vi "LoadFeedforward.vi"(8 "error in":errorcluster, 10 "show ref":refnum<vi>, 11 "Path":path) -> (0 "error out":errorcluster, 2 "values Q":dbl[](array[numeric]), 3 "values I":dbl[](array[numeric]))   [LabVIEW 2013]
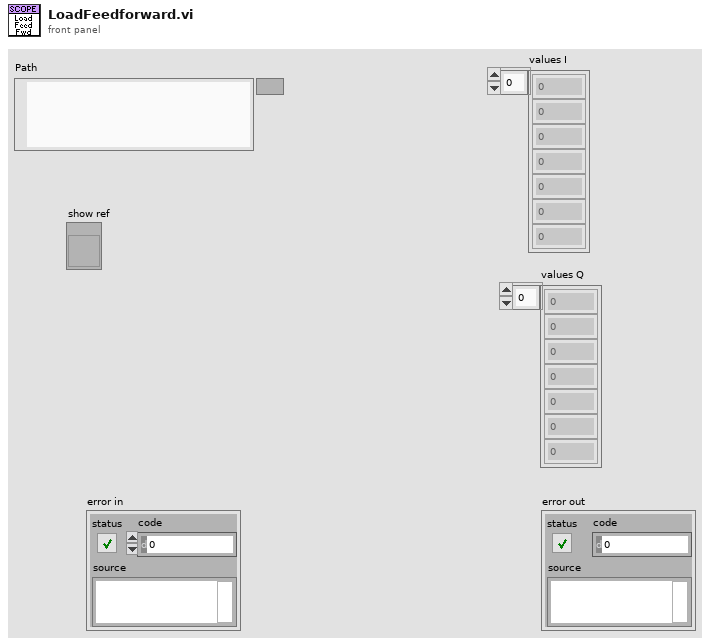
[diagram p1: front panel]
types:
  T1 = enum8{"Enabled", "Disabled", "Disabled and Grayed Out"}
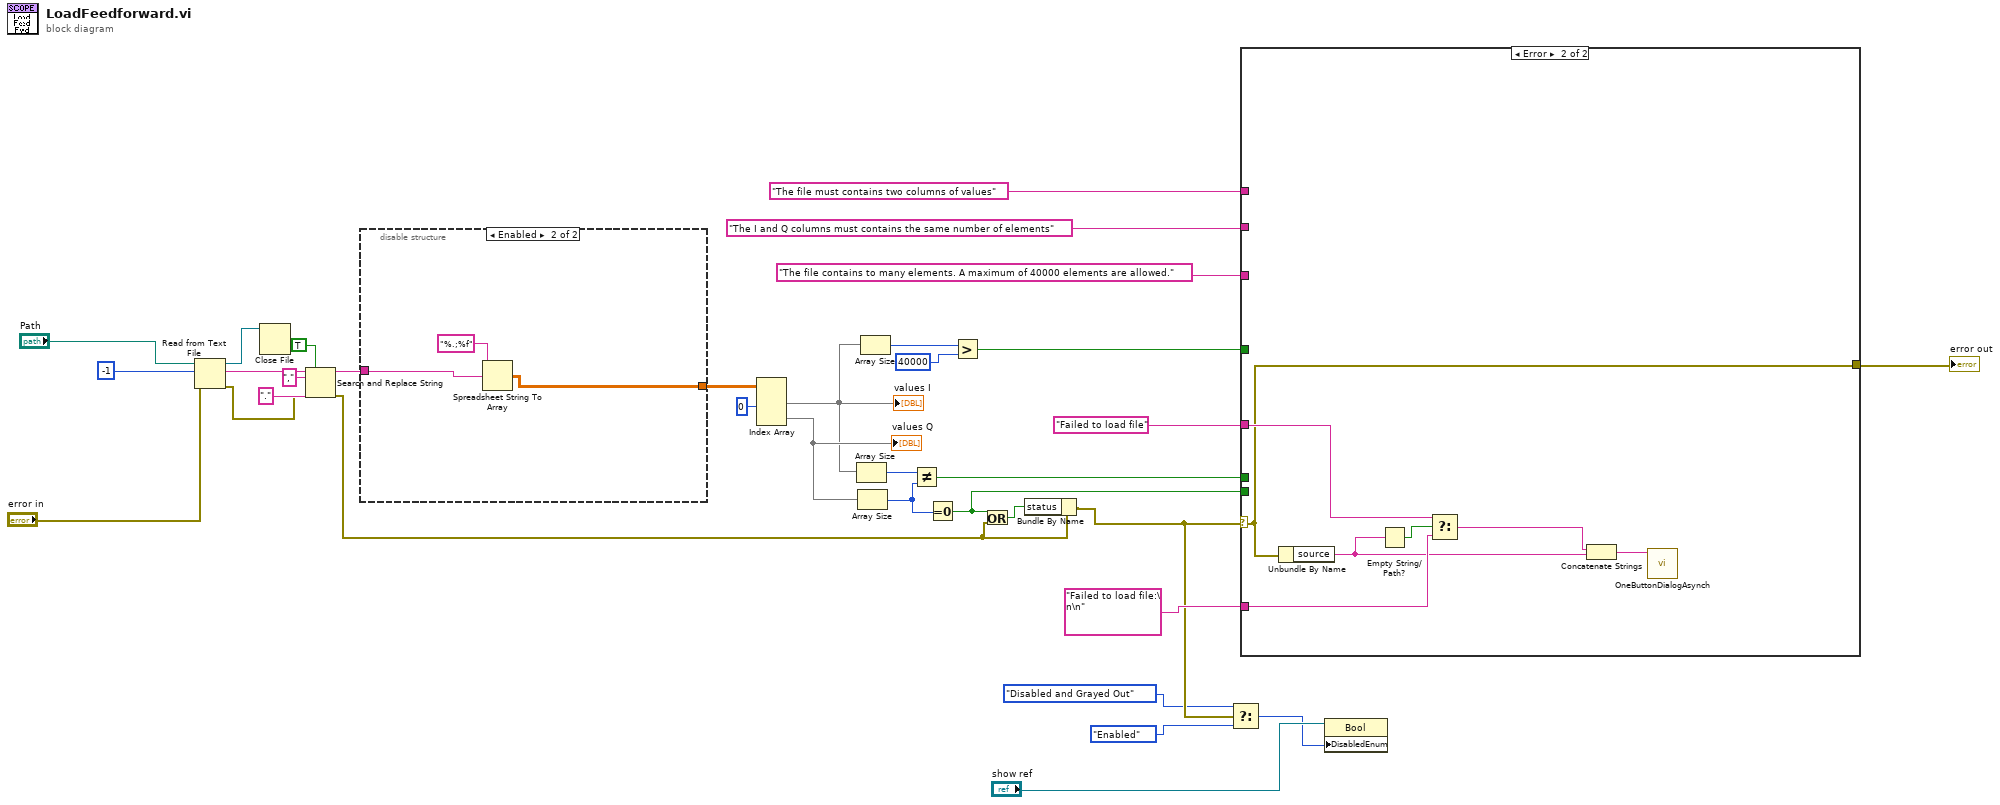
[diagram p0: block diagram]
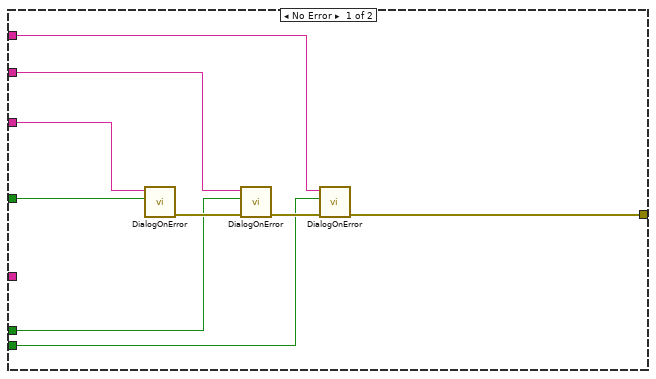
[diagram p2: hidden frame]
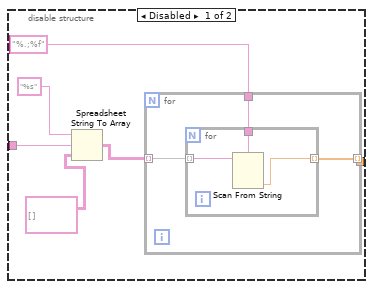
[diagram p3: hidden frame]
diagram:
  n1 = Read from Text File(file (use dialog)="Path", count=-1, error in="error in") -> (refnum out=w32:refnum<file>, text=w31:string, error out=w24:errorcluster)  [unwired: 1 in, 1 out]
  n2 = Close File(refnum=w32) -> ()  [unwired: 1 in, 2 out]
  n3 = Search and Replace String(replace all?=TRUE ("replace all? (F)"), input string=w31, search string=",", replace string="." ("replace string (\"\")"), error in=w24) -> (result string=w26:string, error out=w21:errorcluster)  [unwired: 3 in, 2 out]
  n4 = disable-structure shown="Enabled" {
    disable-tunnel: w26 -> [w36 w47]
    disable-tunnel: [_ w46] -> w25
    frame Disabled {
      n5 = Spreadsheet String To Array(format string="%s", spreadsheet string=w36, array type (2D Dbl)=string[][] []) -> (array=w37:string[][])  [unwired: 1 in]
      n6 = for {
        tunnel: "%.;%f" ("format string") -> [w42]
        tunnel: w37 -> [w41] mode=indexing
        tunnel: [w40] -> _ mode=indexing
        n7 = for {
          tunnel: w42 -> [w45]
          tunnel: w41 -> [w44] mode=indexing
          tunnel: [w43] -> w40 mode=indexing
          n8 = Scan From String(format string=w45, input string=w44) -> (output 1=w43:dbl)  [unwired: 3 in, 3 out]
        }
      }
    }
    frame Enabled {
      n9 = Spreadsheet String To Array(format string="%.;%f", spreadsheet string=w47) -> (array=w46:dbl[][])  [unwired: 2 in]
    }
  }
  n10 = Index Array(array=w25, index (col) #1=0 ("disabled index (col)")) -> (element #1=w10:dbl[], element #2=w11:dbl[])  [unwired: 3 in]
  "values I" <- w10
  "values Q" <- w11
  n11 = Array Size(array=w10) -> (size(s)=w23:i32)
  n12 = Array Size(array=w11) -> (size(s)=w22:i32)
  n13 = Array Size(array=w10) -> (size(s)=w9:i32)
  n14 = Not Equal?(x=w23, y=w22) -> (x != y?=w5:bool)
  n15 = Equal To 0?(x=w22) -> (x = 0?=w4:bool)
  n16 = Greater?(x=w9, y=40000) -> (0:w7:bool)
  n17 = Or(x=w4, y=w21) -> (x .or. y?=w20:bool)
  n18 = Bundle By Name(cluster=w21, "status"=w20) -> (w16:errorcluster)
  n19 = Select(t=T1."Disabled and Grayed Out" ("Disabled"), s=w16, f=T1."Enabled" ("Disabled")) -> (s? t:f=w12:T1)
  n20 = case shown="Error" w16 {
    selector: w16 -> [_ w58]
    tunnel: "Failed to load file:\n\n" -> [_ w62]
    tunnel: "Failed to load file" -> [_ w61]
    tunnel: w7 -> [w57 _]
    tunnel: "The file contains to many elements. A maximum of 40000 elements are allowed." -> [w56 _]
    tunnel: w5 -> [w53 _]
    tunnel: w4 -> [w52 _]
    tunnel: "The I and Q columns must contains the same number of elements" -> [w51 _]
    tunnel: "The file must contains two columns of values" -> [w50 _]
    tunnel: [w49 w58] -> w1
    frame No Error {
      n21 = call "DialogOnError.vi"("Show"=w57, "Message"=w56) -> ("error out"=w55:errorcluster)  [unwired: 9 in]
      n22 = call "DialogOnError.vi"("error in (no error)"=w55, "Show"=w53, "Message"=w51) -> ("error out"=w54:errorcluster)  [unwired: 8 in]
      n23 = call "DialogOnError.vi"("error in (no error)"=w54, "Show"=w52, "Message"=w50) -> ("error out"=w49:errorcluster)  [unwired: 8 in]
    }
    frame Error {
      n24 = Unbundle By Name(w58) -> ("source"=w59:string)
      n25 = Empty String/Path?(string/path=w59) -> (empty?=w63:bool)
      n26 = Select(t=w61, s=w63, f=w62) -> (s? t:f=w60:string)
      n27 = Concatenate Strings(w60, w59) -> (w64:string)
      n28 = call "OneButtonDialogAsynch.vi"("Message to Display"=w64) -> ()  [unwired: 10 in, 1 out]
    }
  }
  "error out" <- w1
  n29 = property class="Bool"(reference="show ref", "DisabledEnum"=w12) -> ()  [unwired: 1 in, 2 out]
